vi "LiftControl.vi"   [LabVIEW 2010]
uses:
  <vilib>/NXT/NXTIO Xnodes/AddressXNode/NXTIOAddress.xnode
  <vilib>/NXT/Subs/MotorXNode.DC Motor Type.ctl
  4150_RingItUp_State/4150 ringbot v1.lvrbt
  <vilib>/NXT/Subs/MotorXNode.2DCMotor.ctl
  <vilib>/NXT/Block Support/NXT_ButtonSelector.ctl
  <vilib>/NXT/Subs/LVHSConnector.ctl
  <vilib>/NXT/NXTIO Xnodes/NXTIOXNode/NXTIO.xnode
  <vilib>/NXT/Dual Mode Library/Sensors/readNXTButton.vi
  <vilib>/NXT/NXTIO Xnodes/NXTIONodeSubVIs/TETRIX IO Move DC Motors.vi
types:
  T1 = enum16{"Initialize", "Idle", "Up", "Down", "Switch Power", "Exit", ""}
  T2 = typedef "MotorXNode.DC Motor Type.ctl" = enum16{"DC Motor"}
  T3 = cluster{"DC Motor":T2, "Address":i16, "Address":i16}
  T4 = typedef "NXT_ButtonSelector.ctl" = u16
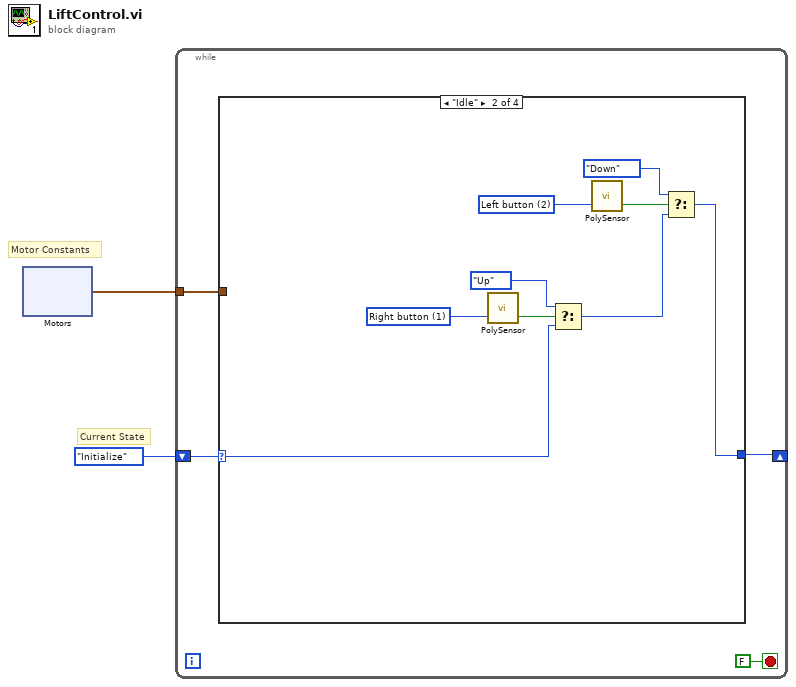
[diagram p0: block diagram]
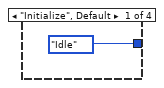
[diagram p2: hidden frame]
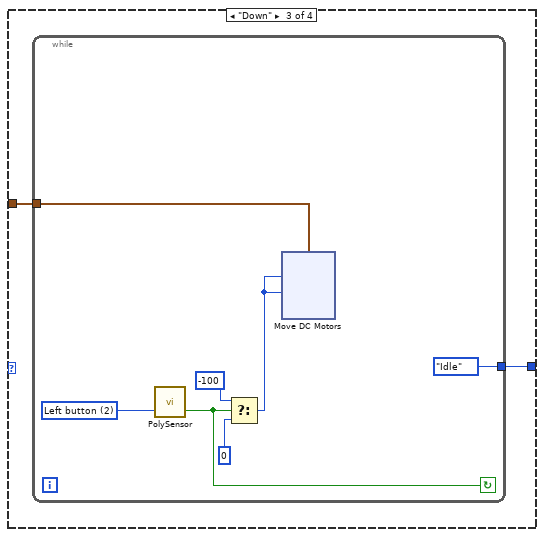
[diagram p3: hidden frame]
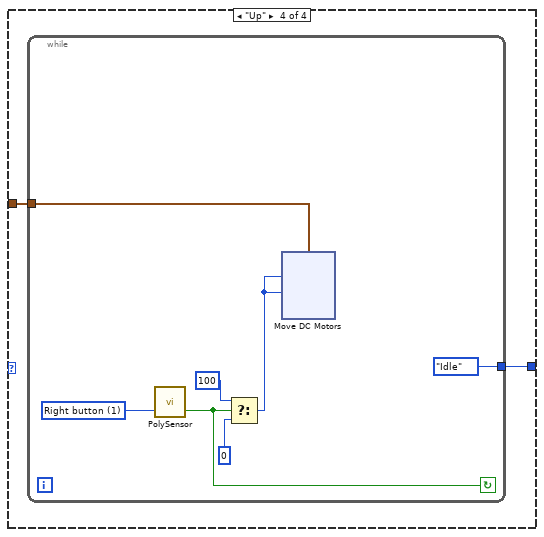
[diagram p4: hidden frame]
diagram:
  # "Current State"
  # "Motor Constants"
  n1 = xnode "Motors"() -> ("DC Motor"=w1:T3)
  n2 = while {
    shift-right: [w4] -> _
    shift-left: T1."Initialize" -> [w6]
    tunnel: w1 -> [w5]
    stop <- FALSE stop-if-true
    n3 = case shown="\"Idle\"" w6 {
      selector: w6 -> [_ w8 _ _]
      tunnel: w5 -> [_ _ w18 w37]
      tunnel: [T1."Idle" w9 w17 w36] -> w4
      frame "Initialize", Default {
      }
      frame "Idle" {
        w15 = T4 2 items=["Enter button"=3, "Left button"=2, "Right button"=1] ("Button (Enter button)")
        w16 = T4 1 items=["Enter button"=3, "Left button"=2, "Right button"=1] ("Button (Enter button)")
        n4 = call-poly <vilib>:"PolySensor.vi"("Button (Enter button)"=w16) -> ("Yes/No"=w11:bool)  [unwired: 2 in, 1 out]
        n5 = Select(t=T1."Up", s=w11, f=w8) -> (s? t:f=w10:T1)
        n6 = call-poly <vilib>:"PolySensor.vi"("Button (Enter button)"=w15) -> ("Yes/No"=w14:bool)  [unwired: 2 in, 1 out]
        n7 = Select(t=T1."Down", s=w14, f=w10) -> (s? t:f=w9:T1)
      }
      frame "Down" {
        n8 = while {
          tunnel: w18 -> [w25]
          tunnel: [T1."Idle"] -> w17
          stop <- w19 continue-if-true
          w23 = T4 2 items=["Enter button"=3, "Left button"=2, "Right button"=1] ("Button (Enter button)")
          n9 = call-poly <vilib>:"PolySensor.vi"("Button (Enter button)"=w23) -> ("Yes/No"=w19:bool)  [unwired: 2 in, 1 out]
          n10 = Select(t=-100, s=w19, f=0) -> (s? t:f=w20:i32)
          n11 = xnode "Move DC Motors"("Power/Speed 2"=w20, "Power/Speed 1"=w20, "Motors"=w25) -> ()  [unwired: 1 in, 1 out]
        }
      }
      frame "Up" {
        n12 = while {
          tunnel: w37 -> [w44]
          tunnel: [T1."Idle"] -> w36
          stop <- w38 continue-if-true
          w42 = T4 1 items=["Enter button"=3, "Left button"=2, "Right button"=1] ("Button (Enter button)")
          n13 = call-poly <vilib>:"PolySensor.vi"("Button (Enter button)"=w42) -> ("Yes/No"=w38:bool)  [unwired: 2 in, 1 out]
          n14 = Select(t=100, s=w38, f=0) -> (s? t:f=w39:i32)
          n15 = xnode "Move DC Motors"("Power/Speed 2"=w39, "Power/Speed 1"=w39, "Motors"=w44) -> ()  [unwired: 1 in, 1 out]
        }
      }
    }
  }
